vi "Thermocouple - SW-Timed Input.vi"() -> ()   [LabVIEW 2020]
doc: "This example demonstrates how to continuously acquire thermocouple measurements using a DAQmx device.\n\nFor instructions on how to connect your signals to the DAQ device, refer to your device documentation."
uses:
  <vilib>/DAQmx/create/channels.llb/DAQmx Create Channel (AI-Temperature-Thermocouple).vi
  <vilib>/DAQmx/miscellaneous.llb/DAQmx Fill In Error Info.vi
  <vilib>/DAQmx/read.llb/DAQmx Read (Analog 1D Wfm NChan 1Samp).vi
  <resource>/objmgr/daqmx.rc
panel:
  in  "Auto Zero Mode":i32(ring)=10230 items=["None"=10230, "Once"=10244, "Every Sample"=10164]
  in  "CJC Channel":refnum<k21>
  in  "CJC Value":dbl=25.0 format="%0.2f"
  in  "CJC Source":i32(ring)=10116 items=["Built-In"=10200, "Constant Value"=10116, "Channel"=10113]
  in  "Thermocouple Type":i32(ring)=10072 items=["J"=10072, "K"=10073, "N"=10077, "R"=10082, "S"=10085, "T"=10086, "B"=10047, "E"=10055]
  in  "Units":i32(ring)=10143 items=["Deg C"=10143, "Deg F"=10144, "Kelvins"=10325, "Deg R"=10145, "From Custom Scale"=10065]
  in  "Loop Time (ms)":u32=100
  in  "Stop":bool
  in  "Max Temperature":dbl=100.0
  in  "Min Temperature":dbl
  in  "Physical Channel":tag="Dev1/ai0"
  out "Waveform Chart":waveform(dbl)[](graph)
  # "Channel Settings"
  # "Acquired Data"
  # "Timing Settings"
  # "Auto Zero Settings"
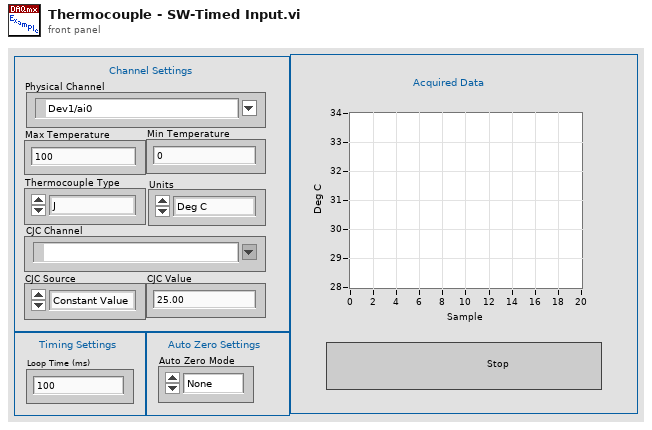
[diagram p1: front panel]
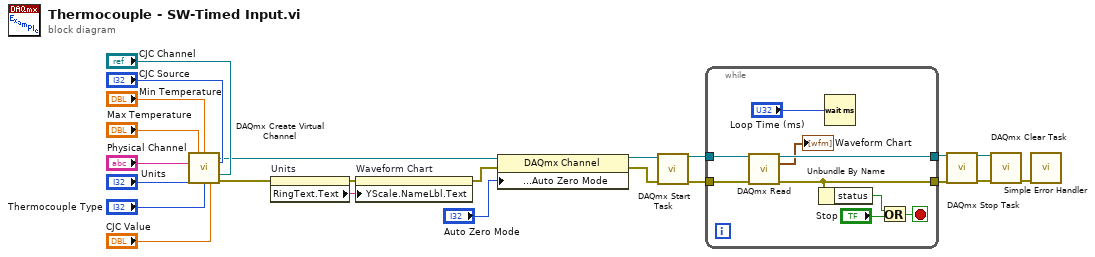
[diagram p0: block diagram]
diagram:
  n1 = call-poly <vilib>:"DAQmx Create Virtual Channel.vi"("maximum value"="Max Temperature", "minimum value"="Min Temperature", "physical channels"="Physical Channel", "cjc source"="CJC Source", "units"="Units", "cjc channel"="CJC Channel", "thermocouple type"="Thermocouple Type", "cjc value"="CJC Value") -> ("task out"=w10:refnum<k21>, "error out"=w12:errorcluster)  [unwired: 6 in]
  n2 = property on="Units" class="Ring (strict)"(error in=w12) -> (error out=w6:errorcluster, "RingText.Text"=w7:string)  [unwired: 1 in, 1 out]
  n3 = property on="Waveform Chart" class="WFChart (strict)"(error in=w6, "YScale.NameLbl.Text"=w7) -> (error out=w5:errorcluster)  [unwired: 1 in, 1 out]
  n4 = property class="DAQmx Channel"(reference=w10, error in=w5, "Analog Input:General Properties:Advanced:High Accuracy Settings:Auto Zero Mode"="Auto Zero Mode") -> (reference out=w9:refnum<k21>, error out=w8:errorcluster)
  n5 = call <vilib>:"DAQmx Start Task.vi"("task/channels in"=w9, "error in"=w8) -> ("task out"=w23:refnum<k21>, "error out"=w22:errorcluster)  [unwired: 12 in]
  n6 = while {
    tunnel: w23 -> [w32]
    tunnel: w22 -> [w31]
    tunnel: [w28] -> w1
    tunnel: [w29] -> w2
    stop <- w30 stop-if-true
    n7 = call-poly <vilib>:"DAQmx Read.vi"("task/channels in"=w32, "error in"=w31) -> ("task out"=w29:refnum<k21>, "data"=→"Waveform Chart":waveform(dbl)[], "error out"=w28:errorcluster)  [unwired: 11 in]
    n8 = Unbundle By Name(w28) -> ("status"=w27:bool)
    n9 = Wait (ms)(milliseconds to wait="Loop Time (ms)") -> ()  [unwired: 1 out]
    n10 = Or(x=w27, y="Stop") -> (x .or. y?=w30:bool)
  }
  n11 = call <vilib>:"DAQmx Stop Task.vi"("task/channels in"=w2, "error in"=w1) -> ("task out"=w4:refnum<k21>, "error out"=w3:errorcluster)  [unwired: 12 in]
  n12 = call <vilib>:"DAQmx Clear Task.vi"("task in"=w4, "error in"=w3) -> ("error out"=w21:errorcluster)  [unwired: 13 in]
  n13 = call <vilib>:"Simple Error Handler.vi"("error in (no error)"=w21) -> ()  [unwired: 4 in, 5 out]
